vi "Apply Numeric Extensions.vi"(8 "error in (no error)":errorcluster, 10 "JSON string in":string, 11 "JSON Serializer in":refnum<class "JSON Serializer.lvclass">) -> (0 "error out":errorcluster, 2 "JSON string out":string, 3 "JSON Serializer out":refnum<class "JSON Serializer.lvclass">)   [LabVIEW 2019, in "JKI JSON Serialization.lvlib" / "JSON Serializer.lvclass"]
doc: "JKI JSON 1.1.10.37\nTomi Maila - JKI\nCopyright (c) 2017, JKI"
uses:
  JSON Serializer.lvclass
  JSON Serializer.lvclass/JSON Serializer.ctl
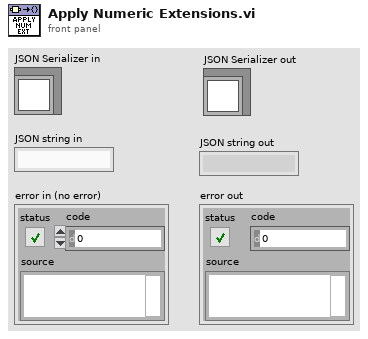
[diagram p1: front panel]
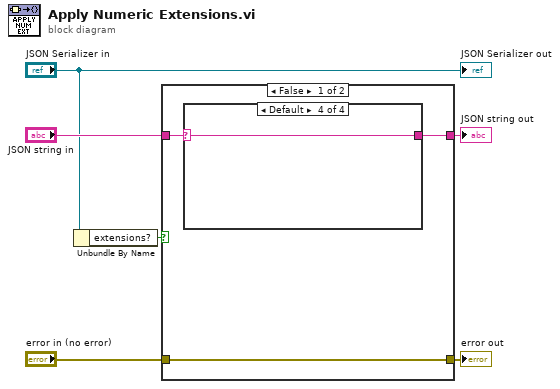
[diagram p0: block diagram]
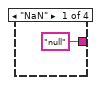
[diagram p2: hidden frame]
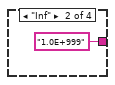
[diagram p3: hidden frame]
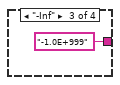
[diagram p4: hidden frame]
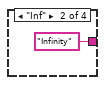
[diagram p7: hidden frame]
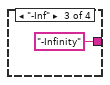
[diagram p8: hidden frame]
diagram:
  n1 = Unbundle By Name("JSON Serializer in") -> ("extensions?"=w4:bool)
  n2 = case shown="False" w4 {
    tunnel: "error in (no error)" -> [w7 w14]
    tunnel: [w7 w14] -> w3
    tunnel: [w8 w15] -> w5
    tunnel: "JSON string in" -> [w9 w16]
    frame False {
      n3 = case shown="Default" w9 {
        selector: w9 -> [_ _ _ w13]
        tunnel: ["null" "1.0E+999" "-1.0E+999" w13] -> w8
        frame "NaN" {
        }
        frame "Inf" {
        }
        frame "-Inf" {
        }
        frame Default {
        }
      }
    }
    frame True {
      n4 = case shown="Default" w16 {
        selector: w16 -> [w17 _ _ w20]
        tunnel: [w17 "Infinity" "-Infinity" w20] -> w15
        frame "NaN" {
        }
        frame "Inf" {
        }
        frame "-Inf" {
        }
        frame Default {
        }
      }
    }
  }
  "JSON string out" <- w5
  "error out" <- w3
  "JSON Serializer out" <- "JSON Serializer in"
